vi "Format Markdown Header.vi"(8 "Error In":errorcluster, 9 "Header Size":T1(ring), 11 "Unformatted Heading Input":string) -> (0 "Error Out":errorcluster, 3 "Formatted Header Output":string)   [LabVIEW 2017]
panel:
  # "Accepts a string, formats string into markdown Header header"
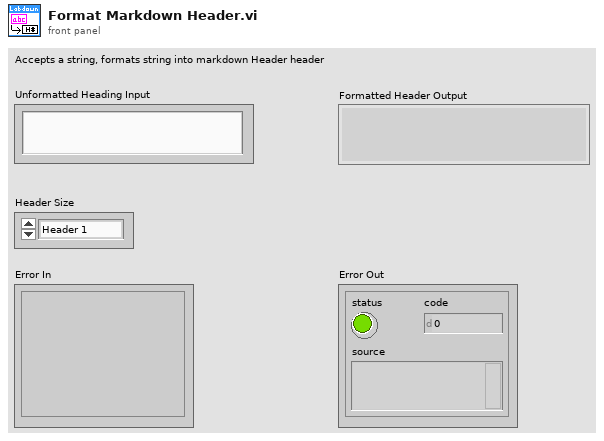
[diagram p1: front panel]
types:
  T1 = enum16{"Header 1", "Header 2", "Header 3", "Header 4", "Header 5", "Header 6"}
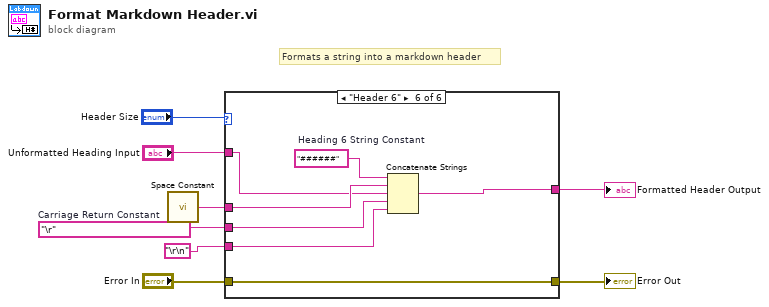
[diagram p0: block diagram]
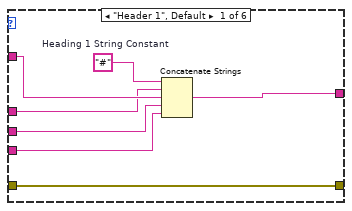
[diagram p2: hidden frame]
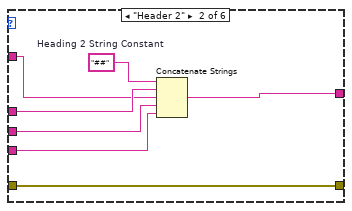
[diagram p3: hidden frame]
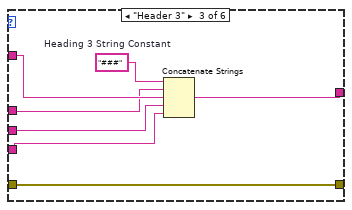
[diagram p4: hidden frame]
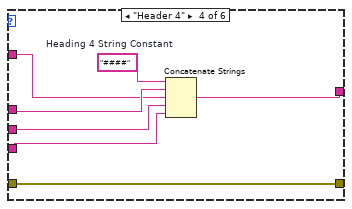
[diagram p5: hidden frame]
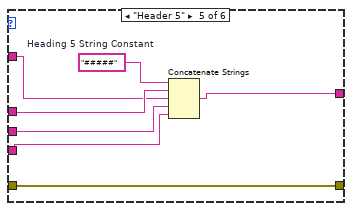
[diagram p6: hidden frame]
diagram:
  w2 = "\r"  # Carriage Return Constant
  # "Formats a string into a markdown header"
  n1 = call <vilib>:"Space Constant.vi"() -> ("String"=w5:string)
  n2 = case shown="\"Header 6\"" "Header Size" {
    tunnel: "Unformatted Heading Input" -> [w14 w20 w28 w34 w41 w48]
    tunnel: [w13 w19 w26 w33 w40 w47] -> w7
    tunnel: w5 -> [w12 w21 w27 w35 w42 w49]
    tunnel: "\r\n" -> [w10 w17 w24 w31 w38 w45]
    tunnel: "Error In" -> [w11 w18 w25 w32 w39 w46]
    tunnel: [w11 w18 w25 w32 w39 w46] -> w3
    tunnel: w2 -> [w9 w16 w23 w30 w37 w44]
    frame "Header 1", Default {
      w15 = "#"  # Heading 1 String Constant
      n3 = Concatenate Strings(w15, w12, w14, w9, w10) -> (w13:string)
    }
    frame "Header 2" {
      w22 = "##"  # Heading 2 String Constant
      n4 = Concatenate Strings(w22, w21, w20, w16, w17) -> (w19:string)
    }
    frame "Header 3" {
      w29 = "###"  # Heading 3 String Constant
      n5 = Concatenate Strings(w29, w27, w28, w23, w24) -> (w26:string)
    }
    frame "Header 4" {
      w36 = "####"  # Heading 4 String Constant
      n6 = Concatenate Strings(w36, w35, w34, w30, w31) -> (w33:string)
    }
    frame "Header 5" {
      w43 = "#####"  # Heading 5 String Constant
      n7 = Concatenate Strings(w43, w42, w41, w37, w38) -> (w40:string)
    }
    frame "Header 6" {
      w50 = "######"  # Heading 6 String Constant
      n8 = Concatenate Strings(w50, w49, w48, w44, w45) -> (w47:string)
    }
  }
  "Formatted Header Output" <- w7
  "Error Out" <- w3
